vi "RDS Serial Handle Frame.vi"(8 "error in (no error)":errorcluster, 10 "RDS Serial Frame":refnum<class "RDS Serial Frame.lvclass">, 11 "Battery Instrument in":refnum<class "Battery Instrument.lvclass">) -> (0 "error out":errorcluster, 3 "Battery Instrument out":refnum<class "Battery Instrument.lvclass">)   [LabVIEW 2015, in "Battery Instrument.lvlib" / "Battery Instrument.lvclass"]
uses:
  Battery Instrument.lvclass
  Libraries/RDS Serial Handler/RDS Serial Frame.lvclass
  Actors/RDS Parent Actor/RDS Parent Actor/RDS Parent Actor.lvclass
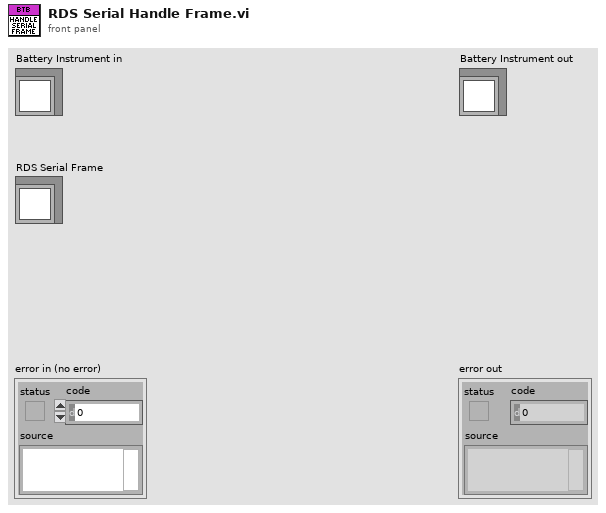
[diagram p1: front panel]
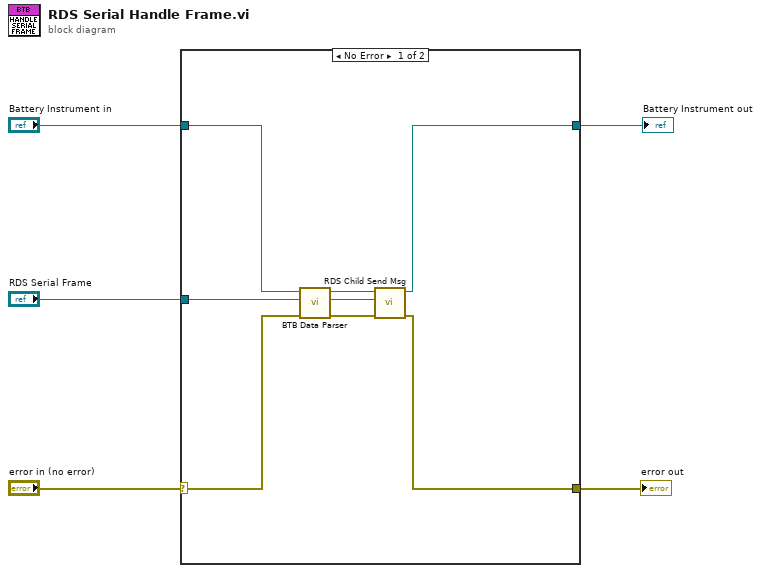
[diagram p0: block diagram]
diagram:
  n1 = case shown="No Error" "error in (no error)" {
    selector: "error in (no error)" -> [w8 w15]
    tunnel: [w6 w15] -> w4
    tunnel: [w9 w14] -> w3
    tunnel: "Battery Instrument in" -> [w13 w14]
    tunnel: "RDS Serial Frame" -> [w12 _]
    frame No Error {
      n2 = call "BTB Data Parser.vi"("error in (no error)"=w8, "RDS Serial Frame in"=w12, "Battery Instrument in"=w13) -> ("error out"=w7:errorcluster, "Battery Message out"=w11:refnum<class "Battery Message.lvclass">, "Battery Instrument out"=w10:refnum<class "Battery Instrument.lvclass">)  [unwired: 6 in]
      n3 = call "RDS Child Send Msg.vi"("error in (no error)"=w7, "RDS Message"=w11, "RDS Parent Actor in"=w10) -> ("error out"=w6:errorcluster, "RDS Parent Actor out"=w9:refnum<class "Battery Instrument.lvclass">)  [unwired: 7 in]
    }
    frame Error {
    }
  }
  "error out" <- w4
  "Battery Instrument out" <- w3
